vi "Media_pressao.vi"(8 "Pressao 2":dbl, 11 "Pressao 1":dbl) -> (0 "Diferenca pressao":dbl, 3 "Pressao media":dbl)   [LabVIEW 2019]
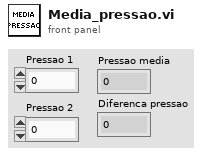
[diagram p1: front panel]
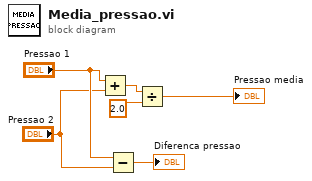
[diagram p0: block diagram]
diagram:
  n1 = Add(x="Pressao 1", y="Pressao 2") -> (x+y=w6:dbl)
  n2 = Subtract(x="Pressao 1", y="Pressao 2") -> (x-y=→"Diferenca pressao":dbl)
  n3 = Divide(x=w6, y=2.0) -> (x/y=→"Pressao media":dbl)
